vi "Begin.vi"(8 "error in":errorcluster) -> (0 "error out":errorcluster)   [LabVIEW 2019]
doc: "Called before other user functions, this VI is expected to open initial I/O refnums, load in file data, and do all program initialization. Notice that the <B>error out</B> terminal is simply used for data flow. Wiring it to other structures or subVIs ensures that this VI runs first."
uses:
  <vilib>/Rock Robotics/WPI/DriverStation/WPI_DriverStationRobotMode2.ctl
  <vilib>/Rock Robotics/WPI/Joystick/WPI_JoystickDeviceEnum.ctl
  <vilib>/Rock Robotics/SystemInterfaces/AI/FPGA_AIChannel.ctl
  <vilib>/Rock Robotics/WPI/ThirdParty/Phoenix-LabVIEW/Motor Controller/Controls/CTRE_Phoenix_MotorControl_NeutralMode.ctl
  <vilib>/Rock Robotics/WPI/ThirdParty/Phoenix-LabVIEW/Motor Controller/Controls/CTRE_Phoenix_MotorControl_ControlMode.ctl
  <vilib>/Rock Robotics/WPI/ThirdParty/Phoenix-LabVIEW/Motor Controller/Controls/CTRE_Phoenix_MotorControl_FeedbackDevice.ctl
  <vilib>/Rock Robotics/WPI/ThirdParty/Phoenix-LabVIEW/Motor Controller/Controls/CTRE_Phoenix_MotorControl_FeedbackDevice_TalonFX.ctl
  <vilib>/Rock Robotics/SystemInterfaces/DIO/FPGA_DIOPWMChannel.ctl
  <vilib>/Rock Robotics/SystemInterfaces/DIO/FPGA_DIOChannel.ctl
  <vilib>/Rock Robotics/WPI/ThirdParty/Phoenix-LabVIEW/Motor Controller/Controls/CTRE_Phoenix_MotorControl_SupplyCurrentLimitConfiguration.ctl
  <vilib>/Rock Robotics/WPI/ThirdParty/Sensors/navX/_TypeDefs/FRIC_navX_DeviceNumbersTypeDef.ctl
  Robot Global Data.vi
  <vilib>/Rock Robotics/WPI/ThirdParty/Phoenix-LabVIEW/Pigeon IMU/CTRE_PigeonIMU_Open_CAN.vi
  <vilib>/Rock Robotics/Network Tables/NT Write Number.vi
  <vilib>/Rock Robotics/WPI/ThirdParty/Phoenix-LabVIEW/Motor Controller/Sensor/CTRE_Phoenix_MotorControl_SetIntegratedSensorPosition_TalonFX.vi
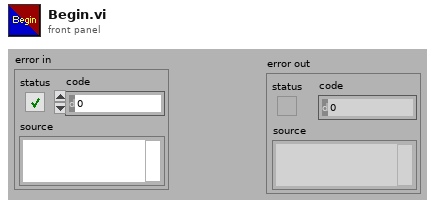
[diagram p1: front panel]
types:
  T1 = typedef "CTRE_Phoenix_MotorControl_SupplyCurrentLimitConfiguration.ctl" = cluster{"Enable?":bool, "Current Limit":dbl, "Threshold Current":dbl, "Threshold Time":dbl}
  T2 = typedef "FRIC_navX_DeviceNumbersTypeDef.ctl" = enum16{"Dev0", "Dev1", "Dev2", "Dev3"}
  T3 = typedef "FPGA_DIOChannel.ctl" = enum8{"DIO 0", "DIO 1", "DIO 2", "DIO 3", "DIO 4", "DIO 5", "DIO 6", "DIO 7", "DIO 8", "DIO 9", "DIO MXP 0", "DIO MXP 1", "DIO MXP 2", "DIO MXP 3", "DIO MXP 4", "DIO MXP 5", "DIO MXP 6", "DIO MXP 7", "DIO MXP 8", "DIO MXP 9", "DIO MXP 10", "DIO MXP 11", "DIO MXP 12", "DIO MXP 13", "DIO MXP 14", "DIO MXP 15", "SPI Port CS1", "SPI Port CS2", "SPI Port CS3", "SPI Port MISO", "SPI Port MOSI", "Invalid"}
  T4 = typedef "FPGA_DIOPWMChannel.ctl" = enum8{"PWM 0", "PWM 1", "PWM 2", "PWM 3", "PWM 4", "PWM 5", "PWM 6", "PWM 7", "PWM 8", "PWM 9", "PWM MXP 0", "PWM MXP 1", "PWM MXP 2", "PWM MXP 3", "PWM MXP 4", "PWM MXP 5", "PWM MXP 6", "PWM MXP 7", "PWM MXP 8", "PWM MXP 9", "Invalid"}
  T5 = typedef "CTRE_Phoenix_MotorControl_NeutralMode.ctl" = enum8{"EEPROMSetting", "Override to Coast", "Override to Brake"}
  T6 = typedef "CTRE_Phoenix_MotorControl_ControlMode.ctl" = u16
  T7 = typedef "CTRE_Phoenix_MotorControl_FeedbackDevice_TalonFX.ctl" = i8
  T8 = typedef "CTRE_Phoenix_MotorControl_FeedbackDevice.ctl" = i8
  T9 = typedef "FPGA_AIChannel.ctl" = enum8{"AI 0", "AI 1", "AI 2", "AI 3", "AI MXP 0", "AI MXP 1", "AI MXP 2", "AI MXP 3", "Invalid"}
  T10 = typedef "WPI_JoystickDeviceEnum.ctl" = enum16{"USB 0", "USB 1", "USB 2", "USB 3", "USB 4", "USB 5"}
  T11 = typedef "WPI_DriverStationRobotMode2.ctl" = enum16{"Autonomous Disabled", "Autonomous Enabled", "Teleop Disabled", "Teleop Enabled", "Disconnected", "Finish", "Test Disabled", "Test Enabled", "Emergency Stopped"}
  T12 = typedef "CTRE_PigeonIMU_DeviceRef.ctl" = cluster{"DeviceStatus":errorcluster, "Device Number":u8, "Type":T13, "Device ID":u32, "Handle":u64, "UsageFrame":u32, "Library Path":path}
  T13 = typedef "CTRE_PigeonIMU_ConnectionType.ctl" = u32
  T14 = typedef "WPI_PotentiometerDevRef.ctl" = cluster{"DevStatus":errorcluster, "Analog Channel":T9, "Invert Output":bool}
  T15 = typedef "WPI_JoystickDevRef.ctl" = cluster{"Device":T10}
  T16 = typedef "WPI_ServoDeviceRef.ctl" = cluster{"DeviceStatus":errorcluster, "PWM Channel":T4, "DeadBand":T17}
  T17 = typedef "WPI_PWMDeadband.ctl" = cluster{"Name":string, "maxPositivePwm":i32, "minPositivePwm":i32, "centerPwm":i32, "maxNegativePwm":i32, "minNegativePwm":i32, "angularRange":u16}
  T18 = typedef "WPI_DigitalInputDevRef.ctl" = cluster{"DevStatus":errorcluster, "DIO Channel":T3}
  T19 = typedef "WPI_MotorControlDeviceRef.ctl" = cluster{"DeviceStatus":errorcluster, "Type":T20, "PWM":cluster{"PWM Channel":T4, "DeadBand":T17}, "CAN":cluster{"Device Number":u8, "SetOutput VI Ref":variant, "GetOutput VI Ref":variant, "Enable VI Ref":variant, "Disable VI Ref":variant, "Data":variant}, "Invert":bool, "DIO PWM":cluster{"PWM \"Enable\" Channel":T4, "DIOChannel":T3, "PWM Rate":dbl}}
  T20 = typedef "WPI_MotorControlType.ctl" = enum16{"PWM", "CAN", "DIO PWM"}
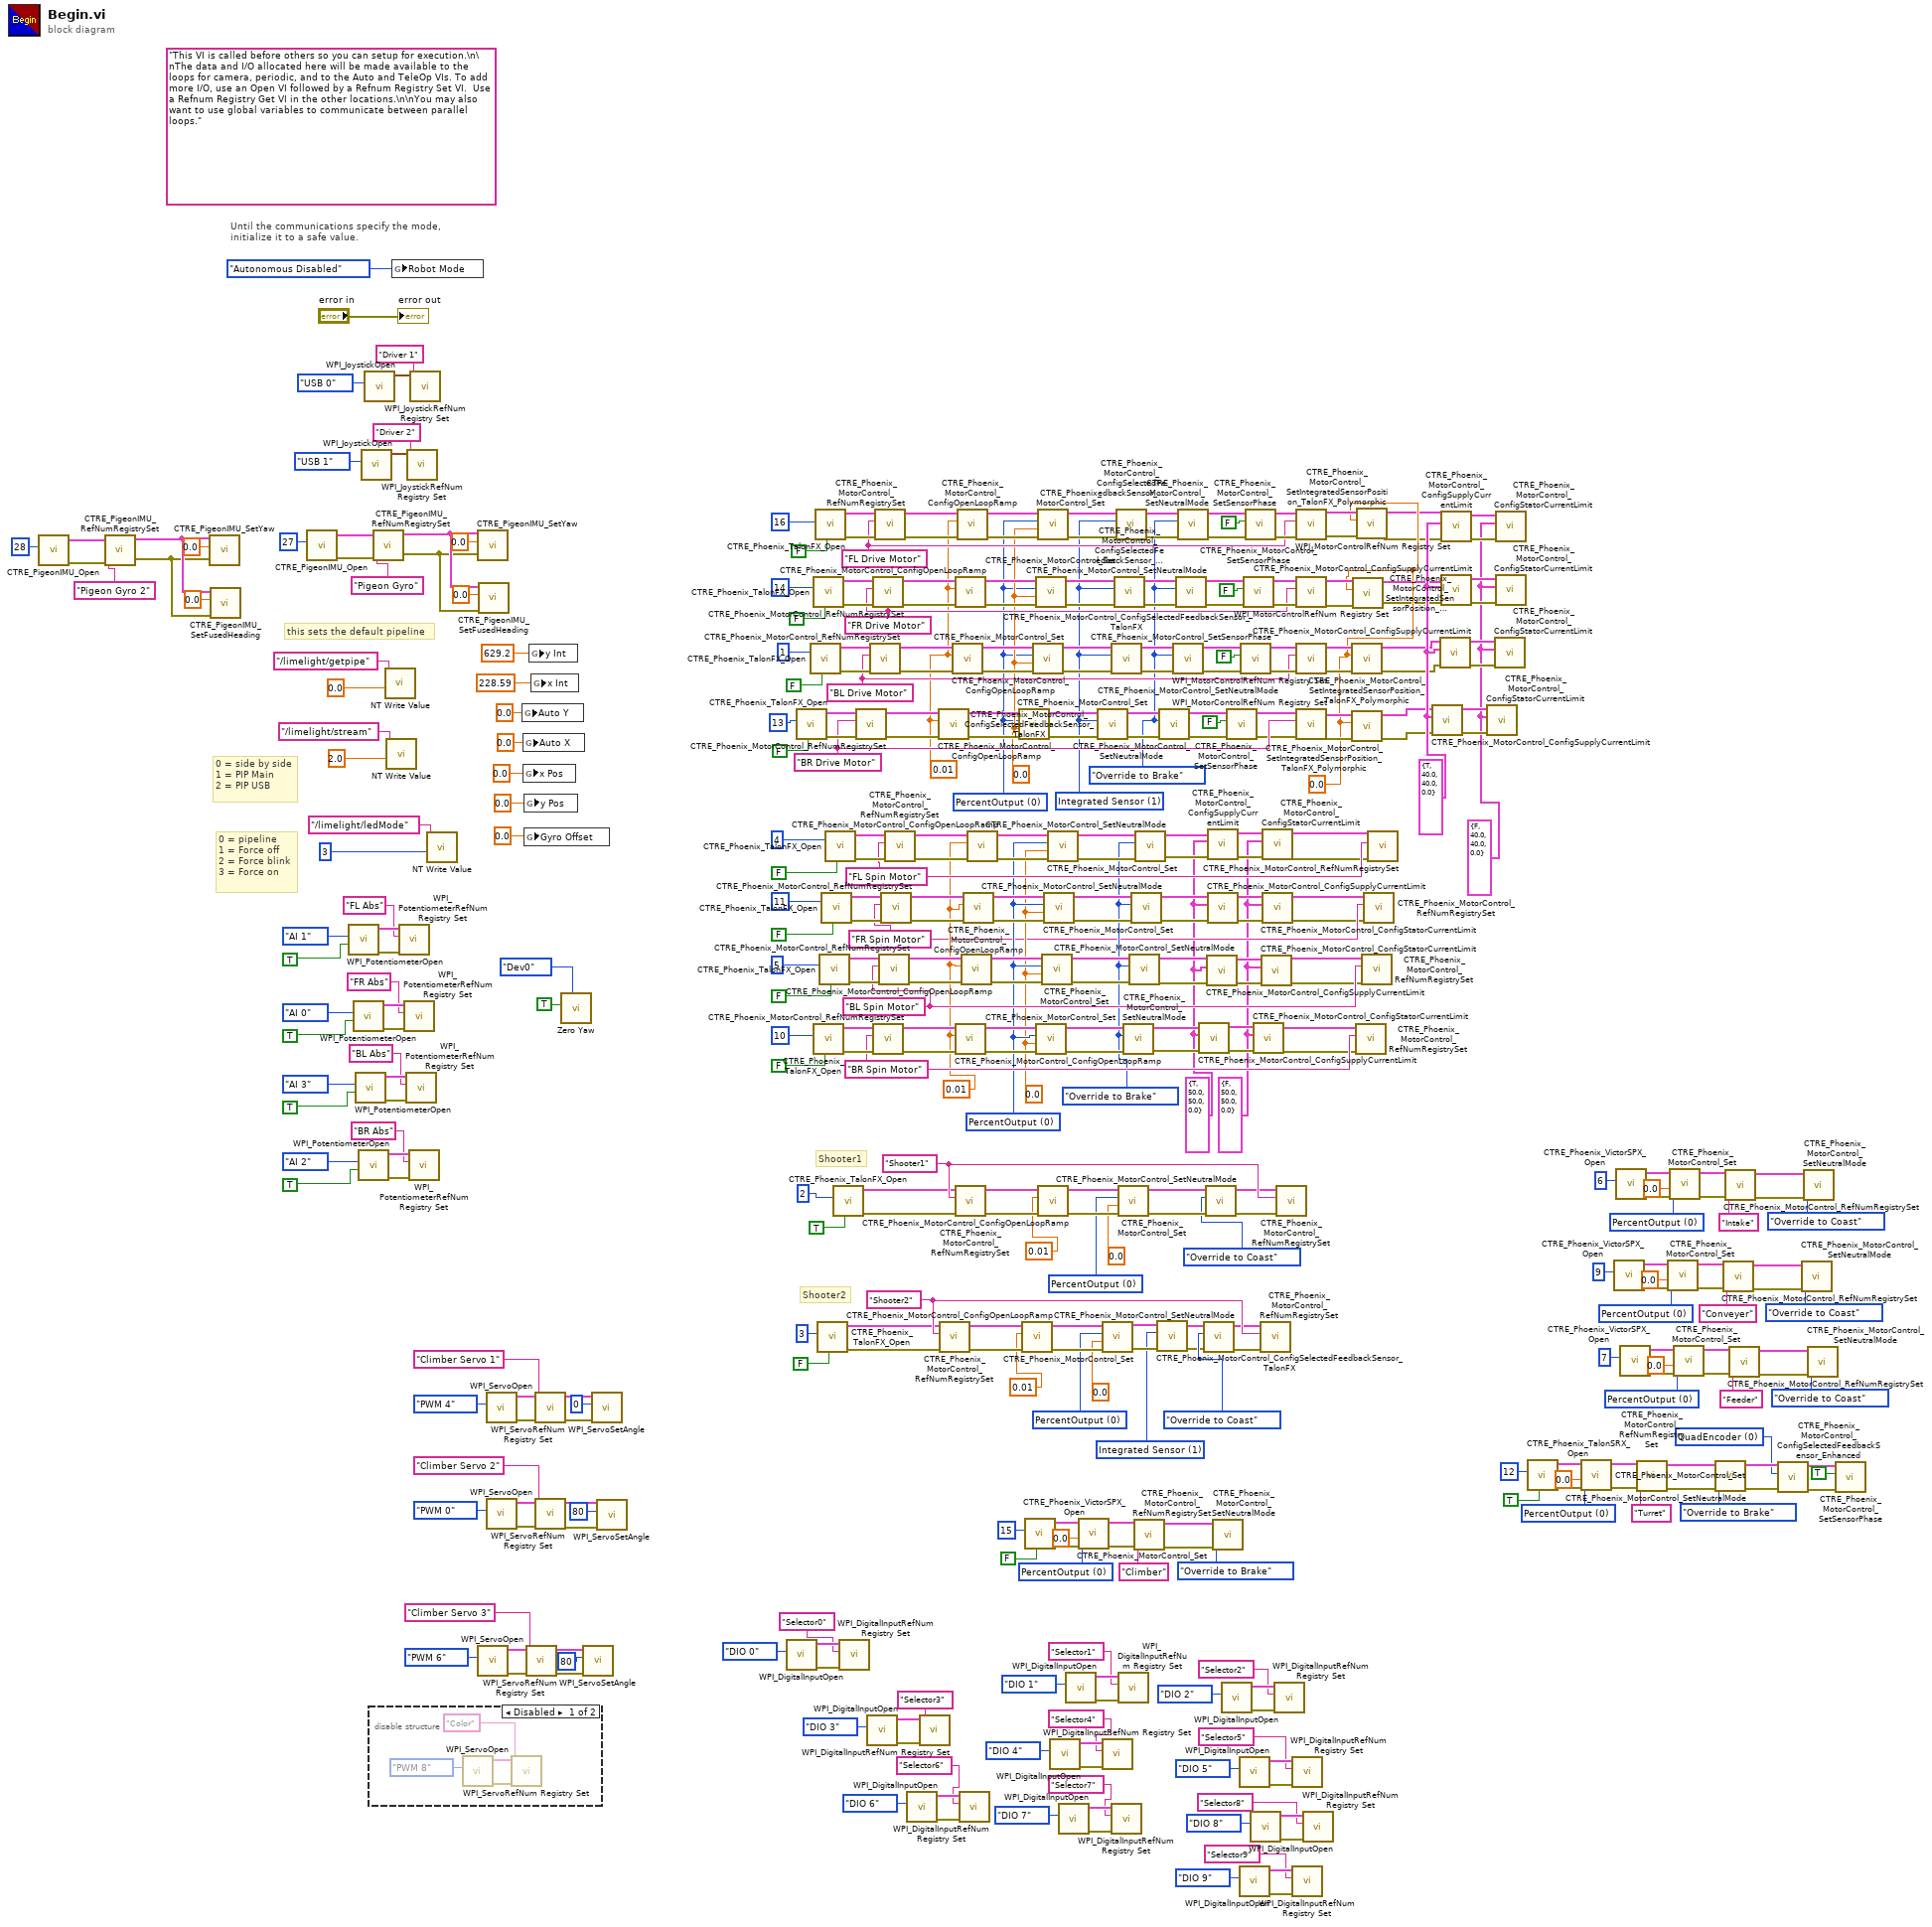
[diagram p0: block diagram]
diagram:
  w1 = T1 {"Enable?"=FALSE, "Current Limit"=50.0, "Threshold Current"=50.0, "Threshold Time"=0.0} ("Supply Current Limit Configuration")
  w2 = T1 {"Enable?"=FALSE, "Current Limit"=40.0, "Threshold Current"=40.0, "Threshold Time"=0.0} ("Supply Current Limit Configuration")
  w14 = T1 {"Enable?"=TRUE, "Current Limit"=40.0, "Threshold Current"=40.0, "Threshold Time"=0.0} ("Supply Current Limit Configuration")
  w23 = T1 {"Enable?"=TRUE, "Current Limit"=50.0, "Threshold Current"=50.0, "Threshold Time"=0.0} ("Supply Current Limit Configuration")
  w92 = 0.0 ("New Position")
  w121 = T6 0 items=["PercentOutput"=0, "Position"=1, "Velocity"=2, "Current"=3, "Follower"=5, "MotionProfile"=6, "MotionMagic"=7, "MotionProfileArc"=10, "Disabled"=15] ("Control Mode")
  w142 = T7 1 items=["Integrated Sensor"=1, "Sensor Sum (S0 + S1)"=9, "Sensor Difference (D0 - D1)"=10, "Remote Source 0"=11, "Remote Source 1"=12, "None"=14, "Software Emulated"=15] ("Talon FX Feedback Device")
  w152 = T8 0 items=["QuadEncoder"=0, "Analog"=2, "Tachometer"=4, "Pulse Width Encoded Position"=8, "Sensor Sum (S0 + S1)"=9, "Sensor Difference (D0 - D1)"=10, "Remote Source 0"=11, "Remote Source 1"=12, "Software Emulated"=15] ("Feedback Device")
  w161 = T6 0 items=["PercentOutput"=0, "Position"=1, "Velocity"=2, "Current"=3, "Follower"=5, "MotionProfile"=6, "MotionMagic"=7, "MotionProfileArc"=10, "Disabled"=15] ("Control Mode")
  w172 = T6 0 items=["PercentOutput"=0, "Position"=1, "Velocity"=2, "Current"=3, "Follower"=5, "MotionProfile"=6, "MotionMagic"=7, "MotionProfileArc"=10, "Disabled"=15] ("Control Mode")
  w169 = "Shooter2" ("refnum name")
  w185 = T6 0 items=["PercentOutput"=0, "Position"=1, "Velocity"=2, "Current"=3, "Follower"=5, "MotionProfile"=6, "MotionMagic"=7, "MotionProfileArc"=10, "Disabled"=15] ("Control Mode")
  w182 = "Shooter1" ("refnum name")
  w205 = T6 0 items=["PercentOutput"=0, "Position"=1, "Velocity"=2, "Current"=3, "Follower"=5, "MotionProfile"=6, "MotionMagic"=7, "MotionProfileArc"=10, "Disabled"=15] ("Control Mode")
  w215 = T6 0 items=["PercentOutput"=0, "Position"=1, "Velocity"=2, "Current"=3, "Follower"=5, "MotionProfile"=6, "MotionMagic"=7, "MotionProfileArc"=10, "Disabled"=15] ("Control Mode")
  w225 = T6 0 items=["PercentOutput"=0, "Position"=1, "Velocity"=2, "Current"=3, "Follower"=5, "MotionProfile"=6, "MotionMagic"=7, "MotionProfileArc"=10, "Disabled"=15] ("Control Mode")
  w253 = CTRE_Phoenix_MotorControl_NeutralMode."Override to Brake" ("Motor Control Neutral Mode")
  w251 = 0.0 ("Output")
  w252 = T6 0 items=["PercentOutput"=0, "Position"=1, "Velocity"=2, "Current"=3, "Follower"=5, "MotionProfile"=6, "MotionMagic"=7, "MotionProfileArc"=10, "Disabled"=15] ("Control Mode")
  w250 = 0.01 ("secondsFromNeutralToFull")
  w297 = CTRE_Phoenix_MotorControl_NeutralMode."Override to Brake" ("Motor Control Neutral Mode")
  w298 = T7 1 items=["Integrated Sensor"=1, "Sensor Sum (S0 + S1)"=9, "Sensor Difference (D0 - D1)"=10, "Remote Source 0"=11, "Remote Source 1"=12, "None"=14, "Software Emulated"=15] ("Talon FX Feedback Device")
  w300 = 0.0 ("Output")
  w299 = T6 0 items=["PercentOutput"=0, "Position"=1, "Velocity"=2, "Current"=3, "Follower"=5, "MotionProfile"=6, "MotionMagic"=7, "MotionProfileArc"=10, "Disabled"=15] ("Control Mode")
  w301 = 0.01 ("secondsFromNeutralToFull")
  w357 = "BR Drive Motor" ("refnum name")
  w302 = "BL Drive Motor" ("refnum name")
  w320 = "FR Drive Motor" ("refnum name")
  w339 = "FL Drive Motor" ("refnum name")
  w254 = "BR Spin Motor" ("refnum name")
  w255 = "BL Spin Motor" ("refnum name")
  w46 = "FR Spin Motor" ("refnum name")
  w256 = "FL Spin Motor" ("refnum name")
  (unwired) "This VI is called before others so you can setup for execution.\n\nThe data and I/O allocated here will be made available to the loops for camera, periodic, and to the Auto and TeleOp VIs. To add more I/O, use an Open VI followed by a Refnum Registry Set VI.  Use a Refnum Registry Get VI in the other locations.\n\nYou may also want to use global variables to communicate between parallel loops."
  # "Shooter2"
  # "Shooter1"
  # "0 = pipeline\n1 = Force off\n2 = Force blink\n3 = Force on"
  # "this sets the default pipeline"
  # "0 = side by side\n1 = PIP Main\n2 = PIP USB"
  # "Until the communications specify the mode,\ninitialize it to a safe value."
  n1 = call-poly <vilib>:"CTRE_PigeonIMU_Open.vi"("Device Number"=u8 28) -> ("error out"=w133:errorcluster, "PigeonIMUDevRef"=w132:T12)  [unwired: 9 in]
  n2 = call <vilib>:"CTRE_PigeonIMU_RefNumRegistrySet.vi"("error in (no error)"=w133, "refnum name"="Pigeon Gyro 2", "PigeonIMUDevRef"=w132) -> ("error out"=w126:errorcluster, "PigeonIMUDevRef"=w129:T12)  [unwired: 7 in]
  n3 = call <vilib>:"CTRE_PigeonIMU_SetYaw.vi"("error in (no error)"=w126, "Value"=0.0, "PigeonIMUDevRef"=w129) -> ()  [unwired: 7 in, 2 out]
  n4 = call <vilib>:"CTRE_PigeonIMU_SetFusedHeading.vi"("error in (no error)"=w126, "Value"=0.0, "PigeonIMUDevRef 2"=w129) -> ()  [unwired: 7 in, 2 out]
  n5 = call-poly <vilib>:"CTRE_PigeonIMU_Open.vi"("Device Number"=u8 27) -> ("error out"=w393:errorcluster, "PigeonIMUDevRef"=w392:T12)  [unwired: 9 in]
  n6 = call <vilib>:"WPI_PotentiometerOpen.vi"("Invert Output"=TRUE, "Analog Channel"=FPGA_AIChannel."AI 1") -> ("error out"=w247:errorcluster, "PotDevRef"=w246:T14)  [unwired: 8 in]
  n7 = call <vilib>:"WPI_PotentiometerOpen.vi"("Invert Output"=TRUE, "Analog Channel"=FPGA_AIChannel."AI 0") -> ("error out"=w242:errorcluster, "PotDevRef"=w241:T14)  [unwired: 8 in]
  n8 = call <vilib>:"WPI_PotentiometerOpen.vi"("Invert Output"=TRUE, "Analog Channel"=FPGA_AIChannel."AI 3") -> ("error out"=w237:errorcluster, "PotDevRef"=w236:T14)  [unwired: 8 in]
  n9 = call <vilib>:"WPI_PotentiometerOpen.vi"("Invert Output"=TRUE, "Analog Channel"=FPGA_AIChannel."AI 2") -> ("error out"=w232:errorcluster, "PotDevRef"=w231:T14)  [unwired: 8 in]
  n10 = call <vilib>:"WPI_JoystickOpen.vi"("JoystickDevice"=WPI_JoystickDeviceEnum."USB 1") -> ("JoystickDevRef"=w385:T15)  [unwired: 10 in]
  n11 = call <vilib>:"WPI_JoystickOpen.vi"("JoystickDevice"=WPI_JoystickDeviceEnum."USB 0") -> ("JoystickDevRef"=w396:T15)  [unwired: 10 in]
  n12 = disable-structure shown="Disabled" {
    frame Disabled {
      n13 = call <vilib>:"WPI_ServoOpen.vi"("PWM Channel"=FPGA_DIOPWMChannel."PWM 8") -> ("error out"=w402:errorcluster, "ServoDeviceRef"=w401:T16)  [unwired: 9 in]
      n14 = call <vilib>:"WPI_ServoRefNum Registry Set.vi"("error in (no error)"=w402, "refnum name"="Color", "ServoDeviceRef"=w401) -> ()  [unwired: 7 in, 2 out]
    }
    frame Enabled {
    }
  }
  n15 = call <vilib>:"CTRE_PigeonIMU_RefNumRegistrySet.vi"("error in (no error)"=w393, "refnum name"="Pigeon Gyro", "PigeonIMUDevRef"=w392) -> ("error out"=w388:errorcluster, "PigeonIMUDevRef"=w389:T12)  [unwired: 7 in]
  n16 = call-poly <vilib>:"NT Write Value.vi"("Numeric"=0.0, "Name"="/limelight/getpipe") -> ()  [unwired: 9 in, 1 out]
  n17 = call-poly <vilib>:"NT Write Value.vi"("Numeric"=2.0, "Name"="/limelight/stream") -> ()  [unwired: 9 in, 1 out]
  n18 = global write "Robot Global Data.vi" "Robot Mode"(WPI_DriverStationRobotMode2."Autonomous Disabled" ("Robot Mode")) -> ()
  n19 = call <vilib>:"WPI_PotentiometerRefNum Registry Set.vi"("error in (no error)"=w247, "refnum name"="FL Abs", "PotDevRef"=w246) -> ()  [unwired: 7 in, 2 out]
  n20 = call <vilib>:"WPI_PotentiometerRefNum Registry Set.vi"("error in (no error)"=w242, "refnum name"="FR Abs", "PotDevRef"=w241) -> ()  [unwired: 7 in, 2 out]
  n21 = call <vilib>:"WPI_PotentiometerRefNum Registry Set.vi"("error in (no error)"=w237, "refnum name"="BL Abs", "PotDevRef"=w236) -> ()  [unwired: 7 in, 2 out]
  n22 = call <vilib>:"WPI_JoystickRefNum Registry Set.vi"("refnum name"="Driver 2", "JoystickDevRef"=w385) -> ()  [unwired: 8 in, 2 out]
  n23 = call <vilib>:"WPI_PotentiometerRefNum Registry Set.vi"("error in (no error)"=w232, "refnum name"="BR Abs", "PotDevRef"=w231) -> ()  [unwired: 7 in, 2 out]
  n24 = call <vilib>:"WPI_JoystickRefNum Registry Set.vi"("refnum name"="Driver 1", "JoystickDevRef"=w396) -> ()  [unwired: 8 in, 2 out]
  n25 = call-poly <vilib>:"NT Write Value.vi"("Numeric"=3, "Name"="/limelight/ledMode") -> ()  [unwired: 9 in, 1 out]
  n26 = call <vilib>:"CTRE_PigeonIMU_SetYaw.vi"("error in (no error)"=w388, "Value"=0.0, "PigeonIMUDevRef"=w389) -> ()  [unwired: 7 in, 2 out]
  n27 = call <vilib>:"WPI_ServoOpen.vi"("PWM Channel"=FPGA_DIOPWMChannel."PWM 6") -> ("error out"=w107:errorcluster, "ServoDeviceRef"=w106:T16)  [unwired: 9 in]
  n28 = call <vilib>:"CTRE_PigeonIMU_SetFusedHeading.vi"("error in (no error)"=w388, "Value"=0.0, "PigeonIMUDevRef 2"=w389) -> ()  [unwired: 7 in, 2 out]
  n29 = call <vilib>:"WPI_ServoOpen.vi"("PWM Channel"=FPGA_DIOPWMChannel."PWM 4") -> ("error out"=w141:errorcluster, "ServoDeviceRef"=w140:T16)  [unwired: 9 in]
  n30 = call <vilib>:"WPI_ServoOpen.vi"("PWM Channel"=FPGA_DIOPWMChannel."PWM 0") -> ("error out"=w137:errorcluster, "ServoDeviceRef"=w136:T16)  [unwired: 9 in]
  n31 = global write "Robot Global Data.vi" "Auto Y"(0.0 ("Auto Y")) -> ()
  n32 = global write "Robot Global Data.vi" "Auto X"(0.0 ("Auto Y")) -> ()
  n33 = global write "Robot Global Data.vi" "x Pos"(0.0 ("Auto Y")) -> ()
  n34 = global write "Robot Global Data.vi" "y Pos"(0.0 ("Auto Y")) -> ()
  n35 = global write "Robot Global Data.vi" "Gyro Offset"(0.0 ("Auto Y")) -> ()
  n36 = call <vilib>:"WPI_ServoRefNum Registry Set.vi"("error in (no error)"=w107, "refnum name"="Climber Servo 3", "ServoDeviceRef"=w106) -> ("error out"=w103:errorcluster, "ServoDeviceRef"=w102:T16)  [unwired: 7 in]
  n37 = global write "Robot Global Data.vi" "y Int"(629.2 ("Auto Y")) -> ()
  n38 = global write "Robot Global Data.vi" "x Int"(228.59 ("Auto Y")) -> ()
  n39 = call <vilib>:"WPI_ServoRefNum Registry Set.vi"("error in (no error)"=w141, "refnum name"="Climber Servo 1", "ServoDeviceRef"=w140) -> ("error out"=w113:errorcluster, "ServoDeviceRef"=w112:T16)  [unwired: 7 in]
  n40 = call <vilib>:"WPI_ServoRefNum Registry Set.vi"("error in (no error)"=w137, "refnum name"="Climber Servo 2", "ServoDeviceRef"=w136) -> ("error out"=w111:errorcluster, "ServoDeviceRef"=w110:T16)  [unwired: 7 in]
  n41 = call <vilib>:"Zero Yaw.vi"("Device Number"=FRIC_navX_DeviceNumbersTypeDef."Dev0", "Zero"=TRUE) -> ()  [unwired: 10 in]
  n42 = call <vilib>:"WPI_ServoSetAngle.vi"("error in (no error)"=w103, "Angle"=80, "ServoDeviceRef"=w102) -> ()  [unwired: 7 in, 2 out]
  n43 = call <vilib>:"WPI_ServoSetAngle.vi"("error in (no error)"=w113, "Angle"=0, "ServoDeviceRef"=w112) -> ()  [unwired: 7 in, 2 out]
  n44 = call <vilib>:"WPI_ServoSetAngle.vi"("error in (no error)"=w111, "Angle"=80, "ServoDeviceRef"=w110) -> ()  [unwired: 7 in, 2 out]
  n45 = call <vilib>:"WPI_DigitalInputOpen.vi"("DIO Channel"=FPGA_DIOChannel."DIO 0") -> ("error out"=w88:errorcluster, "DigitalInputDevRef"=w87:T18)  [unwired: 9 in]
  n46 = call <vilib>:"CTRE_Phoenix_TalonFX_Open.vi"("Invert"=FALSE, "Device Number"=u8 13) -> ("error out"=w373:errorcluster, "CAN Talon SRX Ref"=w372:T19)  [unwired: 8 in]
  n47 = call <vilib>:"CTRE_Phoenix_TalonFX_Open.vi"("Invert"=FALSE, "Device Number"=u8 1) -> ("error out"=w319:errorcluster, "CAN Talon SRX Ref"=w318:T19)  [unwired: 8 in]
  n48 = call <vilib>:"CTRE_Phoenix_TalonFX_Open.vi"("Invert"=FALSE, "Device Number"=u8 14) -> ("error out"=w337:errorcluster, "CAN Talon SRX Ref"=w336:T19)  [unwired: 8 in]
  n49 = call <vilib>:"CTRE_Phoenix_TalonFX_Open.vi"("Invert"=FALSE, "Device Number"=u8 10) -> ("error out"=w269:errorcluster, "CAN Talon SRX Ref"=w268:T19)  [unwired: 8 in]
  n50 = call <vilib>:"CTRE_Phoenix_TalonFX_Open.vi"("Invert"=FALSE, "Device Number"=u8 16) -> ("error out"=w355:errorcluster, "CAN Talon SRX Ref"=w354:T19)  [unwired: 8 in]
  n51 = call <vilib>:"CTRE_Phoenix_TalonFX_Open.vi"("Invert"=FALSE, "Device Number"=u8 3) -> ("error out"=w180:errorcluster, "CAN Talon SRX Ref"=w168:T19)  [unwired: 8 in]
  n52 = call <vilib>:"CTRE_Phoenix_TalonFX_Open.vi"("Invert"=FALSE, "Device Number"=u8 5) -> ("error out"=w278:errorcluster, "CAN Talon SRX Ref"=w277:T19)  [unwired: 8 in]
  n53 = call <vilib>:"CTRE_Phoenix_TalonFX_Open.vi"("Invert"=FALSE, "Device Number"=u8 11) -> ("error out"=w287:errorcluster, "CAN Talon SRX Ref"=w286:T19)  [unwired: 8 in]
  n54 = call <vilib>:"CTRE_Phoenix_TalonFX_Open.vi"("Invert"=FALSE, "Device Number"=u8 4) -> ("error out"=w296:errorcluster, "CAN Talon SRX Ref"=w295:T19)  [unwired: 8 in]
  n55 = call <vilib>:"CTRE_Phoenix_TalonFX_Open.vi"("Invert"=TRUE, "Device Number"=u8 2) -> ("error out"=w196:errorcluster, "CAN Talon SRX Ref"=w181:T19)  [unwired: 8 in]
  n56 = call <vilib>:"WPI_DigitalInputRefNum Registry Set.vi"("error in (no error)"=w88, "refnum name"="Selector0", "DigitalInputDevRef"=w87) -> ()  [unwired: 7 in, 2 out]
  n57 = call <vilib>:"CTRE_Phoenix_MotorControl_RefNumRegistrySet.vi"("error in (no error)"=w373, "refnum name"=w357, "PhoenixMotorControlDevRef"=w372) -> ("error out"=w370:errorcluster, "PhoenixMotorControlDevRef"=w371:T19)  [unwired: 7 in]
  n58 = call <vilib>:"WPI_DigitalInputOpen.vi"("DIO Channel"=FPGA_DIOChannel."DIO 3") -> ("error out"=w84:errorcluster, "DigitalInputDevRef"=w83:T18)  [unwired: 9 in]
  n59 = call <vilib>:"CTRE_Phoenix_MotorControl_RefNumRegistrySet.vi"("error in (no error)"=w319, "refnum name"=w302, "PhoenixMotorControlDevRef"=w318) -> ("error out"=w316:errorcluster, "PhoenixMotorControlDevRef"=w317:T19)  [unwired: 7 in]
  n60 = call <vilib>:"CTRE_Phoenix_MotorControl_RefNumRegistrySet.vi"("error in (no error)"=w337, "refnum name"=w320, "PhoenixMotorControlDevRef"=w336) -> ("error out"=w334:errorcluster, "PhoenixMotorControlDevRef"=w335:T19)  [unwired: 7 in]
  n61 = call <vilib>:"CTRE_Phoenix_MotorControl_RefNumRegistrySet.vi"("error in (no error)"=w269, "refnum name"=w254, "PhoenixMotorControlDevRef"=w268) -> ("error out"=w266:errorcluster, "PhoenixMotorControlDevRef"=w267:T19)  [unwired: 7 in]
  n62 = call <vilib>:"CTRE_Phoenix_MotorControl_RefNumRegistrySet.vi"("error in (no error)"=w355, "refnum name"=w339, "PhoenixMotorControlDevRef"=w354) -> ("error out"=w352:errorcluster, "PhoenixMotorControlDevRef"=w353:T19)  [unwired: 7 in]
  n63 = call <vilib>:"CTRE_Phoenix_MotorControl_RefNumRegistrySet.vi"("error in (no error)"=w278, "refnum name"=w255, "PhoenixMotorControlDevRef"=w277) -> ("error out"=w275:errorcluster, "PhoenixMotorControlDevRef"=w276:T19)  [unwired: 7 in]
  n64 = call <vilib>:"CTRE_Phoenix_MotorControl_RefNumRegistrySet.vi"("error in (no error)"=w287, "refnum name"=w46, "PhoenixMotorControlDevRef"=w286) -> ("error out"=w284:errorcluster, "PhoenixMotorControlDevRef"=w285:T19)  [unwired: 7 in]
  n65 = call <vilib>:"CTRE_Phoenix_MotorControl_RefNumRegistrySet.vi"("error in (no error)"=w296, "refnum name"=w256, "PhoenixMotorControlDevRef"=w295) -> ("error out"=w293:errorcluster, "PhoenixMotorControlDevRef"=w294:T19)  [unwired: 7 in]
  n66 = call <vilib>:"WPI_DigitalInputOpen.vi"("DIO Channel"=FPGA_DIOChannel."DIO 6") -> ("error out"=w81:errorcluster, "DigitalInputDevRef"=w80:T18)  [unwired: 9 in]
  n67 = call <vilib>:"WPI_DigitalInputRefNum Registry Set.vi"("error in (no error)"=w84, "refnum name"="Selector3", "DigitalInputDevRef"=w83) -> ()  [unwired: 7 in, 2 out]
  n68 = call <vilib>:"CTRE_Phoenix_MotorControl_ConfigOpenLoopRamp.vi"("error in (no error)"=w370, "secondsFromNeutralToFull"=w301, "PhoenixMotorControlDevRef"=w371) -> ("error out"=w369:errorcluster, "PhoenixMotorControlDevRef"=w368:T19)  [unwired: 7 in]
  n69 = call <vilib>:"CTRE_Phoenix_MotorControl_RefNumRegistrySet.vi"("error in (no error)"=w180, "refnum name"=w169, "PhoenixMotorControlDevRef"=w168) -> ("error out"=w178:errorcluster, "PhoenixMotorControlDevRef"=w179:T19)  [unwired: 7 in]
  n70 = call <vilib>:"CTRE_Phoenix_MotorControl_ConfigOpenLoopRamp.vi"("error in (no error)"=w316, "secondsFromNeutralToFull"=w301, "PhoenixMotorControlDevRef"=w317) -> ("error out"=w315:errorcluster, "PhoenixMotorControlDevRef"=w314:T19)  [unwired: 7 in]
  n71 = call <vilib>:"CTRE_Phoenix_MotorControl_ConfigOpenLoopRamp.vi"("error in (no error)"=w334, "secondsFromNeutralToFull"=w301, "PhoenixMotorControlDevRef"=w335) -> ("error out"=w333:errorcluster, "PhoenixMotorControlDevRef"=w332:T19)  [unwired: 7 in]
  n72 = call <vilib>:"CTRE_Phoenix_MotorControl_ConfigOpenLoopRamp.vi"("error in (no error)"=w266, "secondsFromNeutralToFull"=w250, "PhoenixMotorControlDevRef"=w267) -> ("error out"=w265:errorcluster, "PhoenixMotorControlDevRef"=w264:T19)  [unwired: 7 in]
  n73 = call <vilib>:"CTRE_Phoenix_MotorControl_RefNumRegistrySet.vi"("error in (no error)"=w196, "refnum name"=w182, "PhoenixMotorControlDevRef"=w181) -> ("error out"=w194:errorcluster, "PhoenixMotorControlDevRef"=w195:T19)  [unwired: 7 in]
  n74 = call <vilib>:"CTRE_Phoenix_MotorControl_ConfigOpenLoopRamp.vi"("error in (no error)"=w352, "secondsFromNeutralToFull"=w301, "PhoenixMotorControlDevRef"=w353) -> ("error out"=w351:errorcluster, "PhoenixMotorControlDevRef"=w350:T19)  [unwired: 7 in]
  n75 = call <vilib>:"WPI_DigitalInputRefNum Registry Set.vi"("error in (no error)"=w81, "refnum name"="Selector6", "DigitalInputDevRef"=w80) -> ()  [unwired: 7 in, 2 out]
  n76 = call <vilib>:"CTRE_Phoenix_MotorControl_ConfigOpenLoopRamp.vi"("error in (no error)"=w275, "secondsFromNeutralToFull"=w250, "PhoenixMotorControlDevRef"=w276) -> ("error out"=w274:errorcluster, "PhoenixMotorControlDevRef"=w273:T19)  [unwired: 7 in]
  n77 = call <vilib>:"CTRE_Phoenix_MotorControl_ConfigOpenLoopRamp.vi"("error in (no error)"=w284, "secondsFromNeutralToFull"=w250, "PhoenixMotorControlDevRef"=w285) -> ("error out"=w283:errorcluster, "PhoenixMotorControlDevRef"=w282:T19)  [unwired: 7 in]
  n78 = call <vilib>:"CTRE_Phoenix_MotorControl_ConfigOpenLoopRamp.vi"("error in (no error)"=w293, "secondsFromNeutralToFull"=w250, "PhoenixMotorControlDevRef"=w294) -> ("error out"=w292:errorcluster, "PhoenixMotorControlDevRef"=w291:T19)  [unwired: 7 in]
  n79 = call <vilib>:"CTRE_Phoenix_MotorControl_Set.vi"("error in (no error)"=w369, "Output"=w300, "Control Mode"=w299, "PhoenixMotorControlDevRef"=w368) -> ("error out"=w367:errorcluster, "PhoenixMotorControlDevRef"=w366:T19)  [unwired: 6 in]
  n80 = call <vilib>:"CTRE_Phoenix_MotorControl_ConfigOpenLoopRamp.vi"("error in (no error)"=w178, "secondsFromNeutralToFull"=0.01, "PhoenixMotorControlDevRef"=w179) -> ("error out"=w177:errorcluster, "PhoenixMotorControlDevRef"=w176:T19)  [unwired: 7 in]
  n81 = call <vilib>:"CTRE_Phoenix_VictorSPX_Open.vi"("Invert"=FALSE, "Device Number"=u8 15) -> ("error out"=w122:errorcluster, "CAN Talon SRX Ref"=w123:T19)  [unwired: 8 in]
  n82 = call <vilib>:"CTRE_Phoenix_MotorControl_Set.vi"("error in (no error)"=w315, "Output"=w300, "Control Mode"=w299, "PhoenixMotorControlDevRef"=w314) -> ("error out"=w313:errorcluster, "PhoenixMotorControlDevRef"=w312:T19)  [unwired: 6 in]
  n83 = call <vilib>:"CTRE_Phoenix_MotorControl_Set.vi"("error in (no error)"=w333, "Output"=w300, "Control Mode"=w299, "PhoenixMotorControlDevRef"=w332) -> ("error out"=w331:errorcluster, "PhoenixMotorControlDevRef"=w330:T19)  [unwired: 6 in]
  n84 = call <vilib>:"CTRE_Phoenix_MotorControl_Set.vi"("error in (no error)"=w265, "Output"=w251, "Control Mode"=w252, "PhoenixMotorControlDevRef"=w264) -> ("error out"=w262:errorcluster, "PhoenixMotorControlDevRef"=w261:T19)  [unwired: 6 in]
  n85 = call <vilib>:"CTRE_Phoenix_MotorControl_Set.vi"("error in (no error)"=w351, "Output"=w300, "Control Mode"=w299, "PhoenixMotorControlDevRef"=w350) -> ("error out"=w349:errorcluster, "PhoenixMotorControlDevRef"=w348:T19)  [unwired: 6 in]
  n86 = call <vilib>:"CTRE_Phoenix_MotorControl_ConfigOpenLoopRamp.vi"("error in (no error)"=w194, "secondsFromNeutralToFull"=0.01, "PhoenixMotorControlDevRef"=w195) -> ("error out"=w193:errorcluster, "PhoenixMotorControlDevRef"=w192:T19)  [unwired: 7 in]
  n87 = call <vilib>:"CTRE_Phoenix_MotorControl_Set.vi"("error in (no error)"=w274, "Output"=w251, "Control Mode"=w252, "PhoenixMotorControlDevRef"=w273) -> ("error out"=w271:errorcluster, "PhoenixMotorControlDevRef"=w270:T19)  [unwired: 6 in]
  n88 = call <vilib>:"CTRE_Phoenix_MotorControl_Set.vi"("error in (no error)"=w283, "Output"=w251, "Control Mode"=w252, "PhoenixMotorControlDevRef"=w282) -> ("error out"=w280:errorcluster, "PhoenixMotorControlDevRef"=w279:T19)  [unwired: 6 in]
  n89 = call <vilib>:"CTRE_Phoenix_MotorControl_Set.vi"("error in (no error)"=w292, "Output"=w251, "Control Mode"=w252, "PhoenixMotorControlDevRef"=w291) -> ("error out"=w289:errorcluster, "PhoenixMotorControlDevRef"=w288:T19)  [unwired: 6 in]
  n90 = call <vilib>:"WPI_DigitalInputOpen.vi"("DIO Channel"=FPGA_DIOChannel."DIO 4") -> ("error out"=w75:errorcluster, "DigitalInputDevRef"=w74:T18)  [unwired: 9 in]
  n91 = call <vilib>:"WPI_DigitalInputOpen.vi"("DIO Channel"=FPGA_DIOChannel."DIO 7") -> ("error out"=w78:errorcluster, "DigitalInputDevRef"=w77:T18)  [unwired: 9 in]
  n92 = call <vilib>:"WPI_DigitalInputOpen.vi"("DIO Channel"=FPGA_DIOChannel."DIO 1") -> ("error out"=w72:errorcluster, "DigitalInputDevRef"=w71:T18)  [unwired: 9 in]
  n93 = call <vilib>:"CTRE_Phoenix_MotorControl_Set.vi"("error in (no error)"=w122, "Output"=0.0, "Control Mode"=w121, "PhoenixMotorControlDevRef"=w123) -> ("error out"=w125:errorcluster, "PhoenixMotorControlDevRef"=w124:T19)  [unwired: 6 in]
  n94 = call <vilib>:"CTRE_Phoenix_MotorControl_ConfigSelectedFeedbackSensor_TalonFX.vi"("error in (no error)"=w367, "Talon FX Feedback Device"=w298, "PhoenixMotorControlDevRef"=w366) -> ("error out"=w365:errorcluster, "PhoenixMotorControlDevRef"=w364:T19)  [unwired: 7 in]
  n95 = call <vilib>:"CTRE_Phoenix_MotorControl_Set.vi"("error in (no error)"=w177, "Output"=0.0, "Control Mode"=w172, "PhoenixMotorControlDevRef"=w176) -> ("error out"=w145:errorcluster, "PhoenixMotorControlDevRef"=w146:T19)  [unwired: 6 in]
  n96 = call <vilib>:"WPI_DigitalInputRefNum Registry Set.vi"("error in (no error)"=w75, "refnum name"="Selector4", "DigitalInputDevRef"=w74) -> ()  [unwired: 7 in, 2 out]
  n97 = call <vilib>:"CTRE_Phoenix_MotorControl_ConfigSelectedFeedbackSensor_TalonFX.vi"("error in (no error)"=w313, "Talon FX Feedback Device"=w298, "PhoenixMotorControlDevRef"=w312) -> ("error out"=w311:errorcluster, "PhoenixMotorControlDevRef"=w310:T19)  [unwired: 7 in]
  n98 = call <vilib>:"WPI_DigitalInputRefNum Registry Set.vi"("error in (no error)"=w78, "refnum name"="Selector7", "DigitalInputDevRef"=w77) -> ()  [unwired: 7 in, 2 out]
  n99 = call <vilib>:"CTRE_Phoenix_MotorControl_ConfigSelectedFeedbackSensor_TalonFX.vi"("error in (no error)"=w331, "Talon FX Feedback Device"=w298, "PhoenixMotorControlDevRef"=w330) -> ("error out"=w329:errorcluster, "PhoenixMotorControlDevRef"=w328:T19)  [unwired: 7 in]
  n100 = call <vilib>:"CTRE_Phoenix_MotorControl_ConfigSelectedFeedbackSensor_TalonFX.vi"("error in (no error)"=w349, "Talon FX Feedback Device"=w298, "PhoenixMotorControlDevRef"=w348) -> ("error out"=w347:errorcluster, "PhoenixMotorControlDevRef"=w346:T19)  [unwired: 7 in]
  n101 = call <vilib>:"CTRE_Phoenix_MotorControl_Set.vi"("error in (no error)"=w193, "Output"=0.0, "Control Mode"=w185, "PhoenixMotorControlDevRef"=w192) -> ("error out"=w190:errorcluster, "PhoenixMotorControlDevRef"=w189:T19)  [unwired: 6 in]
  n102 = call <vilib>:"WPI_DigitalInputRefNum Registry Set.vi"("error in (no error)"=w72, "refnum name"="Selector1", "DigitalInputDevRef"=w71) -> ()  [unwired: 7 in, 2 out]
  n103 = call <vilib>:"CTRE_Phoenix_MotorControl_SetNeutralMode.vi"("error in (no error)"=w262, "Motor Control Neutral Mode"=w253, "PhoenixMotorControlDevRef"=w261) -> ("error out"=w32:errorcluster, "PhoenixMotorControlDevRef"=w33:T19)  [unwired: 7 in]
  n104 = call <vilib>:"CTRE_Phoenix_MotorControl_SetNeutralMode.vi"("error in (no error)"=w271, "Motor Control Neutral Mode"=w253, "PhoenixMotorControlDevRef"=w270) -> ("error out"=w34:errorcluster, "PhoenixMotorControlDevRef"=w35:T19)  [unwired: 7 in]
  n105 = call <vilib>:"CTRE_Phoenix_MotorControl_SetNeutralMode.vi"("error in (no error)"=w280, "Motor Control Neutral Mode"=w253, "PhoenixMotorControlDevRef"=w279) -> ("error out"=w37:errorcluster, "PhoenixMotorControlDevRef"=w36:T19)  [unwired: 7 in]
  n106 = call <vilib>:"CTRE_Phoenix_MotorControl_RefNumRegistrySet.vi"("error in (no error)"=w125, "refnum name"="Climber", "PhoenixMotorControlDevRef"=w124) -> ("error out"=w118:errorcluster, "PhoenixMotorControlDevRef"=w117:T19)  [unwired: 7 in]
  n107 = call <vilib>:"CTRE_Phoenix_MotorControl_SetNeutralMode.vi"("error in (no error)"=w289, "Motor Control Neutral Mode"=w253, "PhoenixMotorControlDevRef"=w288) -> ("error out"=w38:errorcluster, "PhoenixMotorControlDevRef"=w39:T19)  [unwired: 7 in]
  n108 = call <vilib>:"CTRE_Phoenix_MotorControl_ConfigSelectedFeedbackSensor_TalonFX.vi"("error in (no error)"=w145, "Talon FX Feedback Device"=w142, "PhoenixMotorControlDevRef"=w146) -> ("error out"=w144:errorcluster, "PhoenixMotorControlDevRef"=w143:T19)  [unwired: 7 in]
  n109 = call <vilib>:"CTRE_Phoenix_MotorControl_SetNeutralMode.vi"("error in (no error)"=w365, "Motor Control Neutral Mode"=w297, "PhoenixMotorControlDevRef"=w364) -> ("error out"=w363:errorcluster, "PhoenixMotorControlDevRef"=w362:T19)  [unwired: 7 in]
  n110 = call <vilib>:"CTRE_Phoenix_MotorControl_SetNeutralMode.vi"("error in (no error)"=w311, "Motor Control Neutral Mode"=w297, "PhoenixMotorControlDevRef"=w310) -> ("error out"=w309:errorcluster, "PhoenixMotorControlDevRef"=w308:T19)  [unwired: 7 in]
  n111 = call <vilib>:"CTRE_Phoenix_MotorControl_SetNeutralMode.vi"("error in (no error)"=w329, "Motor Control Neutral Mode"=w297, "PhoenixMotorControlDevRef"=w328) -> ("error out"=w327:errorcluster, "PhoenixMotorControlDevRef"=w326:T19)  [unwired: 7 in]
  n112 = call <vilib>:"CTRE_Phoenix_MotorControl_SetNeutralMode.vi"("error in (no error)"=w347, "Motor Control Neutral Mode"=w297, "PhoenixMotorControlDevRef"=w346) -> ("error out"=w345:errorcluster, "PhoenixMotorControlDevRef"=w344:T19)  [unwired: 7 in]
  n113 = call <vilib>:"CTRE_Phoenix_MotorControl_ConfigSupplyCurrentLimit.vi"("error in (no error)"=w32, "Supply Current Limit Configuration"=w23, "PhoenixMotorControlDevRef"=w33) -> ("error out"=w41:errorcluster, "PhoenixMotorControlDevRef"=w40:T19)  [unwired: 7 in]
  n114 = call <vilib>:"CTRE_Phoenix_MotorControl_SetNeutralMode.vi"("error in (no error)"=w144, "Motor Control Neutral Mode"=CTRE_Phoenix_MotorControl_NeutralMode."Override to Coast", "PhoenixMotorControlDevRef"=w143) -> ("error out"=w174:errorcluster, "PhoenixMotorControlDevRef"=w167:T19)  [unwired: 7 in]
  n115 = call <vilib>:"CTRE_Phoenix_MotorControl_SetNeutralMode.vi"("error in (no error)"=w190, "Motor Control Neutral Mode"=CTRE_Phoenix_MotorControl_NeutralMode."Override to Coast", "PhoenixMotorControlDevRef"=w189) -> ("error out"=w187:errorcluster, "PhoenixMotorControlDevRef"=w166:T19)  [unwired: 7 in]
  n116 = call <vilib>:"CTRE_Phoenix_MotorControl_ConfigSupplyCurrentLimit.vi"("error in (no error)"=w34, "Supply Current Limit Configuration"=w23, "PhoenixMotorControlDevRef"=w35) -> ("error out"=w43:errorcluster, "PhoenixMotorControlDevRef"=w42:T19)  [unwired: 7 in]
  n117 = call <vilib>:"CTRE_Phoenix_MotorControl_ConfigSupplyCurrentLimit.vi"("error in (no error)"=w38, "Supply Current Limit Configuration"=w23, "PhoenixMotorControlDevRef"=w39) -> ("error out"=w48:errorcluster, "PhoenixMotorControlDevRef"=w47:T19)  [unwired: 7 in]
  n118 = call <vilib>:"CTRE_Phoenix_MotorControl_ConfigSupplyCurrentLimit.vi"("error in (no error)"=w37, "Supply Current Limit Configuration"=w23, "PhoenixMotorControlDevRef"=w36) -> ("error out"=w45:errorcluster, "PhoenixMotorControlDevRef"=w44:T19)  [unwired: 7 in]
  n119 = call <vilib>:"CTRE_Phoenix_MotorControl_SetNeutralMode.vi"("error in (no error)"=w118, "Motor Control Neutral Mode"=CTRE_Phoenix_MotorControl_NeutralMode."Override to Brake", "PhoenixMotorControlDevRef"=w117) -> ()  [unwired: 7 in, 2 out]
  n120 = call <vilib>:"WPI_DigitalInputOpen.vi"("DIO Channel"=FPGA_DIOChannel."DIO 2") -> ("error out"=w69:errorcluster, "DigitalInputDevRef"=w68:T18)  [unwired: 9 in]
  n121 = call <vilib>:"CTRE_Phoenix_MotorControl_SetSensorPhase.vi"("error in (no error)"=w363, "PhaseSensor"=FALSE, "PhoenixMotorControlDevRef"=w362) -> ("error out"=w356:errorcluster, "PhoenixMotorControlDevRef"=w358:T19)  [unwired: 7 in]
  n122 = call <vilib>:"WPI_DigitalInputOpen.vi"("DIO Channel"=FPGA_DIOChannel."DIO 5") -> ("error out"=w66:errorcluster, "DigitalInputDevRef"=w65:T18)  [unwired: 9 in]
  n123 = call <vilib>:"WPI_DigitalInputOpen.vi"("DIO Channel"=FPGA_DIOChannel."DIO 9") -> ("error out"=w60:errorcluster, "DigitalInputDevRef"=w59:T18)  [unwired: 9 in]
  n124 = call <vilib>:"CTRE_Phoenix_MotorControl_SetSensorPhase.vi"("error in (no error)"=w309, "PhaseSensor"=FALSE, "PhoenixMotorControlDevRef"=w308) -> ("error out"=w304:errorcluster, "PhoenixMotorControlDevRef"=w305:T19)  [unwired: 7 in]
  n125 = call <vilib>:"CTRE_Phoenix_MotorControl_SetSensorPhase.vi"("error in (no error)"=w327, "PhaseSensor"=FALSE, "PhoenixMotorControlDevRef"=w326) -> ("error out"=w322:errorcluster, "PhoenixMotorControlDevRef"=w323:T19)  [unwired: 7 in]
  n126 = call <vilib>:"CTRE_Phoenix_MotorControl_SetSensorPhase.vi"("error in (no error)"=w345, "PhaseSensor"=FALSE, "PhoenixMotorControlDevRef"=w344) -> ("error out"=w340:errorcluster, "PhoenixMotorControlDevRef"=w341:T19)  [unwired: 7 in]
  n127 = call <vilib>:"WPI_DigitalInputOpen.vi"("DIO Channel"=FPGA_DIOChannel."DIO 8") -> ("error out"=w63:errorcluster, "DigitalInputDevRef"=w62:T18)  [unwired: 9 in]
  n128 = call <vilib>:"CTRE_Phoenix_MotorControl_ConfigStatorCurrentLimit.vi"("error in (no error)"=w41, "Stator Current Limit Configuration"=w1, "PhoenixMotorControlDevRef"=w40) -> ("error out"=w24:errorcluster, "PhoenixMotorControlDevRef"=w25:T19)  [unwired: 7 in]
  n129 = call <vilib>:"CTRE_Phoenix_MotorControl_RefNumRegistrySet.vi"("error in (no error)"=w174, "refnum name"=w169, "PhoenixMotorControlDevRef"=w167) -> ()  [unwired: 7 in, 2 out]
  n130 = call <vilib>:"CTRE_Phoenix_MotorControl_ConfigStatorCurrentLimit.vi"("error in (no error)"=w43, "Stator Current Limit Configuration"=w1, "PhoenixMotorControlDevRef"=w42) -> ("error out"=w26:errorcluster, "PhoenixMotorControlDevRef"=w27:T19)  [unwired: 7 in]
  n131 = call <vilib>:"CTRE_Phoenix_MotorControl_ConfigStatorCurrentLimit.vi"("error in (no error)"=w48, "Stator Current Limit Configuration"=w1, "PhoenixMotorControlDevRef"=w47) -> ("error out"=w30:errorcluster, "PhoenixMotorControlDevRef"=w31:T19)  [unwired: 7 in]
  n132 = call <vilib>:"CTRE_Phoenix_MotorControl_ConfigStatorCurrentLimit.vi"("error in (no error)"=w45, "Stator Current Limit Configuration"=w1, "PhoenixMotorControlDevRef"=w44) -> ("error out"=w28:errorcluster, "PhoenixMotorControlDevRef"=w29:T19)  [unwired: 7 in]
  n133 = call <vilib>:"WPI_DigitalInputRefNum Registry Set.vi"("error in (no error)"=w69, "refnum name"="Selector2", "DigitalInputDevRef"=w68) -> ()  [unwired: 7 in, 2 out]
  n134 = call <vilib>:"CTRE_Phoenix_MotorControl_RefNumRegistrySet.vi"("error in (no error)"=w187, "refnum name"=w182, "PhoenixMotorControlDevRef"=w166) -> ()  [unwired: 7 in, 2 out]
  n135 = call <vilib>:"WPI_DigitalInputRefNum Registry Set.vi"("error in (no error)"=w66, "refnum name"="Selector5", "DigitalInputDevRef"=w65) -> ()  [unwired: 7 in, 2 out]
  n136 = call <vilib>:"WPI_DigitalInputRefNum Registry Set.vi"("error in (no error)"=w60, "refnum name"="Selector9", "DigitalInputDevRef"=w59) -> ()  [unwired: 7 in, 2 out]
  n137 = call <vilib>:"WPI_MotorControlRefNum Registry Set.vi"("error in (no error)"=w340, "refnum name"=w339, "MotorControlDevRef"=w341) -> ("error out"=w99:errorcluster, "MotorControlDevRef"=w100:T19)  [unwired: 7 in]
  n138 = call <vilib>:"WPI_MotorControlRefNum Registry Set.vi"("error in (no error)"=w322, "refnum name"=w320, "MotorControlDevRef"=w323) -> ("error out"=w97:errorcluster, "MotorControlDevRef"=w98:T19)  [unwired: 7 in]
  n139 = call <vilib>:"WPI_MotorControlRefNum Registry Set.vi"("error in (no error)"=w304, "refnum name"=w302, "MotorControlDevRef"=w305) -> ("error out"=w95:errorcluster, "MotorControlDevRef"=w96:T19)  [unwired: 7 in]
  n140 = call <vilib>:"WPI_MotorControlRefNum Registry Set.vi"("error in (no error)"=w356, "refnum name"=w357, "MotorControlDevRef"=w358) -> ("error out"=w93:errorcluster, "MotorControlDevRef"=w94:T19)  [unwired: 7 in]
  n141 = call <vilib>:"WPI_DigitalInputRefNum Registry Set.vi"("error in (no error)"=w63, "refnum name"="Selector8", "DigitalInputDevRef"=w62) -> ()  [unwired: 7 in, 2 out]
  n142 = call-poly <vilib>:"CTRE_Phoenix_MotorControl_SetIntegratedSensorPosition_TalonFX_Polymorphic.vi"("error in (no error)"=w95, "New Position"=w92, "PhoenixMotorControlDevRef"=w96) -> ("error out"=w8:errorcluster, "PhoenixMotorControlDevRef"=w9:T19)  [unwired: 7 in]
  n143 = call-poly <vilib>:"CTRE_Phoenix_MotorControl_SetIntegratedSensorPosition_TalonFX_Polymorphic.vi"("error in (no error)"=w93, "New Position"=w92, "PhoenixMotorControlDevRef"=w94) -> ("error out"=w6:errorcluster, "PhoenixMotorControlDevRef"=w7:T19)  [unwired: 7 in]
  n144 = call-poly <vilib>:"CTRE_Phoenix_MotorControl_SetIntegratedSensorPosition_TalonFX_Polymorphic.vi"("error in (no error)"=w97, "New Position"=w92, "PhoenixMotorControlDevRef"=w98) -> ("error out"=w10:errorcluster, "PhoenixMotorControlDevRef"=w11:T19)  [unwired: 7 in]
  n145 = call <vilib>:"CTRE_Phoenix_MotorControl_RefNumRegistrySet.vi"("error in (no error)"=w24, "refnum name"=w254, "PhoenixMotorControlDevRef"=w25) -> ()  [unwired: 7 in, 2 out]
  n146 = call-poly <vilib>:"CTRE_Phoenix_MotorControl_SetIntegratedSensorPosition_TalonFX_Polymorphic.vi"("error in (no error)"=w99, "New Position"=w92, "PhoenixMotorControlDevRef"=w100) -> ("error out"=w12:errorcluster, "PhoenixMotorControlDevRef"=w13:T19)  [unwired: 7 in]
  n147 = call <vilib>:"CTRE_Phoenix_MotorControl_RefNumRegistrySet.vi"("error in (no error)"=w26, "refnum name"=w255, "PhoenixMotorControlDevRef"=w27) -> ()  [unwired: 7 in, 2 out]
  n148 = call <vilib>:"CTRE_Phoenix_MotorControl_RefNumRegistrySet.vi"("error in (no error)"=w28, "refnum name"=w46, "PhoenixMotorControlDevRef"=w29) -> ()  [unwired: 7 in, 2 out]
  n149 = call <vilib>:"CTRE_Phoenix_MotorControl_RefNumRegistrySet.vi"("error in (no error)"=w30, "refnum name"=w256, "PhoenixMotorControlDevRef"=w31) -> ()  [unwired: 7 in, 2 out]
  n150 = call <vilib>:"CTRE_Phoenix_MotorControl_ConfigSupplyCurrentLimit.vi"("error in (no error)"=w6, "Supply Current Limit Configuration"=w14, "PhoenixMotorControlDevRef"=w7) -> ("error out"=w16:errorcluster, "PhoenixMotorControlDevRef"=w15:T19)  [unwired: 7 in]
  n151 = call <vilib>:"CTRE_Phoenix_MotorControl_ConfigSupplyCurrentLimit.vi"("error in (no error)"=w8, "Supply Current Limit Configuration"=w14, "PhoenixMotorControlDevRef"=w9) -> ("error out"=w18:errorcluster, "PhoenixMotorControlDevRef"=w17:T19)  [unwired: 7 in]
  n152 = call <vilib>:"CTRE_Phoenix_MotorControl_ConfigSupplyCurrentLimit.vi"("error in (no error)"=w12, "Supply Current Limit Configuration"=w14, "PhoenixMotorControlDevRef"=w13) -> ("error out"=w22:errorcluster, "PhoenixMotorControlDevRef"=w21:T19)  [unwired: 7 in]
  n153 = call <vilib>:"CTRE_Phoenix_MotorControl_ConfigSupplyCurrentLimit.vi"("error in (no error)"=w10, "Supply Current Limit Configuration"=w14, "PhoenixMotorControlDevRef"=w11) -> ("error out"=w20:errorcluster, "PhoenixMotorControlDevRef"=w19:T19)  [unwired: 7 in]
  n154 = call <vilib>:"CTRE_Phoenix_MotorControl_ConfigStatorCurrentLimit.vi"("error in (no error)"=w16, "Stator Current Limit Configuration"=w2, "PhoenixMotorControlDevRef"=w15) -> ()  [unwired: 7 in, 2 out]
  n155 = call <vilib>:"CTRE_Phoenix_MotorControl_ConfigStatorCurrentLimit.vi"("error in (no error)"=w18, "Stator Current Limit Configuration"=w2, "PhoenixMotorControlDevRef"=w17) -> ()  [unwired: 7 in, 2 out]
  n156 = call <vilib>:"CTRE_Phoenix_MotorControl_ConfigStatorCurrentLimit.vi"("error in (no error)"=w22, "Stator Current Limit Configuration"=w2, "PhoenixMotorControlDevRef"=w21) -> ()  [unwired: 7 in, 2 out]
  n157 = call <vilib>:"CTRE_Phoenix_MotorControl_ConfigStatorCurrentLimit.vi"("error in (no error)"=w20, "Stator Current Limit Configuration"=w2, "PhoenixMotorControlDevRef"=w19) -> ()  [unwired: 7 in, 2 out]
  n158 = call <vilib>:"CTRE_Phoenix_TalonSRX_Open.vi"("Invert"=TRUE, "Device Number"=u8 12) -> ("error out"=w162:errorcluster, "CAN Talon SRX Ref"=w163:T19)  [unwired: 8 in]
  n159 = call <vilib>:"CTRE_Phoenix_MotorControl_Set.vi"("error in (no error)"=w162, "Output"=0.0, "Control Mode"=w161, "PhoenixMotorControlDevRef"=w163) -> ("error out"=w165:errorcluster, "PhoenixMotorControlDevRef"=w164:T19)  [unwired: 6 in]
  n160 = call <vilib>:"CTRE_Phoenix_VictorSPX_Open.vi"("Device Number"=u8 9) -> ("error out"=w216:errorcluster, "CAN Talon SRX Ref"=w217:T19)  [unwired: 9 in]
  n161 = call <vilib>:"CTRE_Phoenix_VictorSPX_Open.vi"("Device Number"=u8 6) -> ("error out"=w226:errorcluster, "CAN Talon SRX Ref"=w227:T19)  [unwired: 9 in]
  n162 = call <vilib>:"CTRE_Phoenix_VictorSPX_Open.vi"("Device Number"=u8 7) -> ("error out"=w206:errorcluster, "CAN Talon SRX Ref"=w207:T19)  [unwired: 9 in]
  n163 = call <vilib>:"CTRE_Phoenix_MotorControl_RefNumRegistrySet.vi"("error in (no error)"=w165, "refnum name"="Turret", "PhoenixMotorControlDevRef"=w164) -> ("error out"=w158:errorcluster, "PhoenixMotorControlDevRef"=w157:T19)  [unwired: 7 in]
  n164 = call <vilib>:"CTRE_Phoenix_MotorControl_Set.vi"("error in (no error)"=w216, "Output"=0.0, "Control Mode"=w215, "PhoenixMotorControlDevRef"=w217) -> ("error out"=w219:errorcluster, "PhoenixMotorControlDevRef"=w218:T19)  [unwired: 6 in]
  n165 = call <vilib>:"CTRE_Phoenix_MotorControl_Set.vi"("error in (no error)"=w226, "Output"=0.0, "Control Mode"=w225, "PhoenixMotorControlDevRef"=w227) -> ("error out"=w229:errorcluster, "PhoenixMotorControlDevRef"=w228:T19)  [unwired: 6 in]
  n166 = call <vilib>:"CTRE_Phoenix_MotorControl_Set.vi"("error in (no error)"=w206, "Output"=0.0, "Control Mode"=w205, "PhoenixMotorControlDevRef"=w207) -> ("error out"=w209:errorcluster, "PhoenixMotorControlDevRef"=w208:T19)  [unwired: 6 in]
  n167 = call <vilib>:"CTRE_Phoenix_MotorControl_SetNeutralMode.vi"("error in (no error)"=w158, "Motor Control Neutral Mode"=CTRE_Phoenix_MotorControl_NeutralMode."Override to Brake", "PhoenixMotorControlDevRef"=w157) -> ("error out"=w154:errorcluster, "PhoenixMotorControlDevRef"=w153:T19)  [unwired: 7 in]
  n168 = call <vilib>:"CTRE_Phoenix_MotorControl_RefNumRegistrySet.vi"("error in (no error)"=w219, "refnum name"="Conveyer", "PhoenixMotorControlDevRef"=w218) -> ("error out"=w212:errorcluster, "PhoenixMotorControlDevRef"=w211:T19)  [unwired: 7 in]
  n169 = call <vilib>:"CTRE_Phoenix_MotorControl_RefNumRegistrySet.vi"("error in (no error)"=w229, "refnum name"="Intake", "PhoenixMotorControlDevRef"=w228) -> ("error out"=w222:errorcluster, "PhoenixMotorControlDevRef"=w221:T19)  [unwired: 7 in]
  n170 = call <vilib>:"CTRE_Phoenix_MotorControl_RefNumRegistrySet.vi"("error in (no error)"=w209, "refnum name"="Feeder", "PhoenixMotorControlDevRef"=w208) -> ("error out"=w202:errorcluster, "PhoenixMotorControlDevRef"=w201:T19)  [unwired: 7 in]
  n171 = call <vilib>:"CTRE_Phoenix_MotorControl_ConfigSelectedFeedbackSensor_Enhanced.vi"("error in (no error)"=w154, "Feedback Device"=w152, "PhoenixMotorControlDevRef"=w153) -> ("error out"=w150:errorcluster, "PhoenixMotorControlDevRef"=w149:T19)  [unwired: 7 in]
  n172 = call <vilib>:"CTRE_Phoenix_MotorControl_SetNeutralMode.vi"("error in (no error)"=w212, "Motor Control Neutral Mode"=CTRE_Phoenix_MotorControl_NeutralMode."Override to Coast", "PhoenixMotorControlDevRef"=w211) -> ()  [unwired: 7 in, 2 out]
  n173 = call <vilib>:"CTRE_Phoenix_MotorControl_SetNeutralMode.vi"("error in (no error)"=w222, "Motor Control Neutral Mode"=CTRE_Phoenix_MotorControl_NeutralMode."Override to Coast", "PhoenixMotorControlDevRef"=w221) -> ()  [unwired: 7 in, 2 out]
  n174 = call <vilib>:"CTRE_Phoenix_MotorControl_SetNeutralMode.vi"("error in (no error)"=w202, "Motor Control Neutral Mode"=CTRE_Phoenix_MotorControl_NeutralMode."Override to Coast", "PhoenixMotorControlDevRef"=w201) -> ()  [unwired: 7 in, 2 out]
  n175 = call <vilib>:"CTRE_Phoenix_MotorControl_SetSensorPhase.vi"("error in (no error)"=w150, "PhaseSensor"=TRUE, "PhoenixMotorControlDevRef"=w149) -> ()  [unwired: 7 in, 2 out]
  "error out" <- "error in"
